vi "Get One Status Test.vi"() -> ()   [LabVIEW 2018, in "AltonTech MALT200817.lvlib"]
doc: "Use this template to build a user interface event handler design pattern. Use this pattern for dialog boxes and other user interfaces. You also can create and execute user-defined events that the VI can handle the same way as user interface events."
uses:
  AltonTech MALT200817.lvlib
  Public/Types/MALT CardTypes.ctl
panel:
  in  "MALT CardType":T1=enum."MALT132"
  in  "Port":i32=1
  in  "Address":i32=3
  out "Status":bool
  out "Cycle":i32
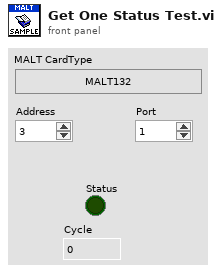
[diagram p1: front panel]
types:
  T1 = typedef "AltonTech MALT200817.lvlib/MALT CardTypes.ctl" = enum32{"-", "YAV90832", "YAV904X8", "MALT132", "YAV91616", "YAV90PIN", "YAV90096", "YAV90HVT", "YAV90CLR", "YAV90128", "YAV90PNE", "YAVCANCON", "YAV91775", "YAV90XXX", "YAV90MMU", "H730050", "H710060", "H710061", "YAV90304", "MMI", "YAV90060", "MALT160T", "YAV90059", "Not Defined"}
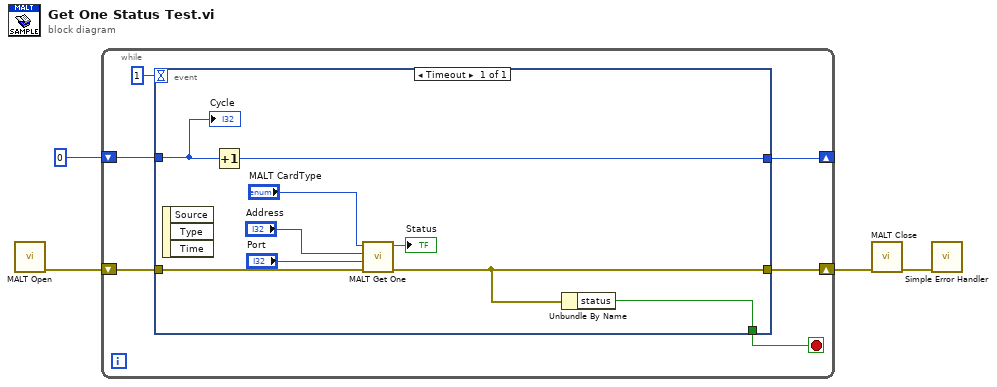
[diagram p0: block diagram]
diagram:
  n1 = call "MALT Open.vi"() -> ("error out"=w4:errorcluster)  [unwired: 11 in]
  n2 = while {
    shift-right: [w7] -> w3
    shift-left: w4 -> [w8]
    shift-right: [w5] -> _
    shift-left: 0 -> [w6]
    stop <- w10 stop-if-true
    n3 = event shown="[0] Timeout" {
      selector: _ -> [_]
      dyn-events: _ -> [_]
      timeout: 1 -> [_]
      tunnel: [w17] -> w10
      tunnel: w8 -> [w19]
      tunnel: [w18] -> w7
      tunnel: w6 -> [w14]
      tunnel: [w13] -> w5
      event Timeout {
        n4 = event-data() -> ()  [unwired: 1 in, 3 out]
        n5 = Increment(x=w14) -> (x+1=w13:i32)
        n6 = call "MALT Get One.vi"("error in"=w19, "Port"="Port", "Address"="Address", "MALT FamilyCode"="MALT CardType") -> ("error out"=w18:errorcluster, "Status"=→"Status":bool)  [unwired: 6 in]
        n7 = Unbundle By Name(w18) -> ("status"=w17:bool)
        "Cycle" <- w14
      }
    }
  }
  n8 = call "MALT Close.vi"("error in"=w3) -> ("error out"=w1:errorcluster)  [unwired: 10 in]
  n9 = call <vilib>:"Simple Error Handler.vi"("error in (no error)"=w1) -> ()  [unwired: 4 in, 5 out]
